vi "SST_Query.vi"(0 "System no.":i32=1 min=1 max=4 step=1, 2 "Axes to query":string[](array[string]), 3 "All axes?":bool, 4 "Axis identifier?":bool=TRUE, 5 "error in":errorcluster) -> (14 "Step size":dbl[](array[numeric]) format="%.6f", 19 "error out":errorcluster)   [LabVIEW 2020]
doc: "Returns step-size setting (e.g. for manual control pad, see also \"SST.vi\").\n\nC-702, C-867, C-880, E-871, E-873: If All axes = TRUE, then Axis identifier can be FALSE\n\nC-887, F-206, M-8X0: All axes = TRUE, Axis identifier = FALSE. Only values for axes X,Y,Z,U,V,W are valid"
panel:
  # "Returns step-size setting (e.g. for manual control pad, see also \"SST.vi\")."
  # "If all axes: use"
  # "Query"
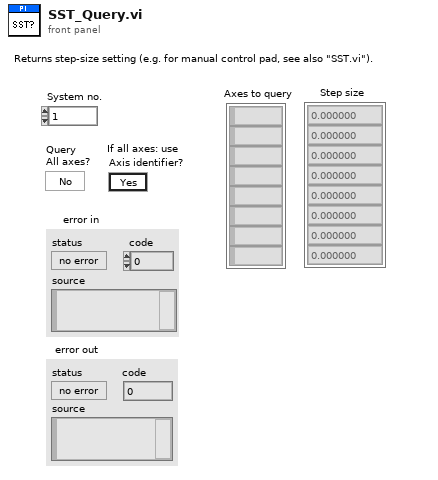
[diagram p1: front panel]
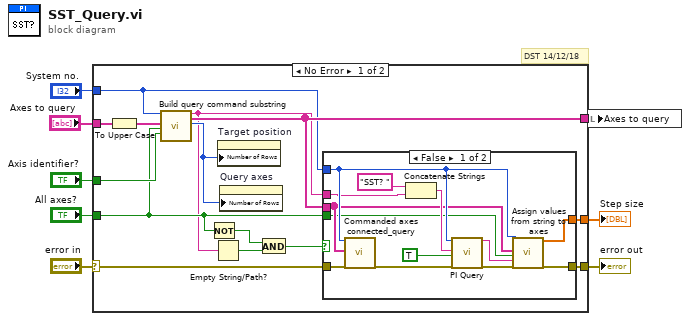
[diagram p0: block diagram]
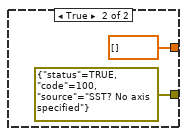
[diagram p2: hidden frame]
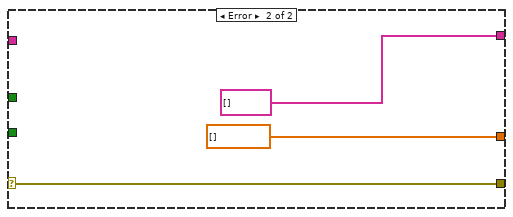
[diagram p3: hidden frame]
diagram:
  # "DST 14/12/18"
  n1 = case shown="No Error" "error in" {
    selector: "error in" -> [w10 w38]
    tunnel: [w22 dbl[] [] ("Values")] -> w8
    tunnel: "Axes to query" -> [w21 _]
    tunnel: [w20 w38] -> w6
    tunnel: "Axis identifier?" -> [w18 _]
    tunnel: "System no." -> [w9 _]
    tunnel: [w16 string[] [] ("Axes to query out")] -> w3
    tunnel: "All axes?" -> [w15 _]
    frame No Error {
      n2 = To Upper Case(1:w21) -> (0:w19:string[])
      n3 = call "Build query command substring.vi"("System no."=w9, "Axes to query in"=w19, "Query\nAll axes?"=w15, "For all axes: use\nAxis identifier?"=w18) -> ("Command substring"=w13:string, "Axes to query out"=w16:string[], "Number of rows"=w17:u32)  [unwired: 2 in, 11 out]
      n4 = Not(x=w15) -> (.not. x?=w14:bool)
      n5 = Empty String/Path?(string/path=w13) -> (empty?=w12:bool)
      n6 = property on="Target position" class="Arr (strict)"("Number of Rows"=w17) -> ()  [unwired: 2 in, 2 out]
      n7 = property on="Query axes" class="Arr (strict)"("Number of Rows"=w17) -> ()  [unwired: 2 in, 2 out]
      n8 = And(x=w14, y=w12) -> (x .and. y?=w11:bool)
      n9 = case shown="False" w11 {
        tunnel: [w32 dbl[] [] ("Values")] -> w22
        tunnel: w10 -> [w31 _]
        tunnel: [w27 errorcluster {"status"=TRUE, "code"=100, "source"="SST? No axis specified"} ("error out")] -> w20
        tunnel: w9 -> [w30 _]
        tunnel: w16 -> [w29 _]
        tunnel: w15 -> [w28 _]
        tunnel: w13 -> [w23 _]
        frame False {
          n10 = call "Commanded axes connected_query.vi"("System no."=w30, "Commanded axes"=w29, "error in"=w31) -> ("error out"=w26:errorcluster)  [unwired: 1 in, 15 out]
          n11 = Concatenate Strings("SST? ", w23) -> (w33:string)
          n12 = call "PI Query.vi"("System no."=w30, "String to send"=w33, "Attach termination char.?"=TRUE ("Attach Linefeed?"), "error in"=w26) -> ("String read"=w25:string, "error out"=w24:errorcluster)  [unwired: 3 in, 11 out]
          n13 = call "Assign values from string to axes.vi"("System no."=w30, "Queried axes"=w29, "All axes queried?"=w28, "Input String"=w25, "error in"=w24) -> ("Values"=w32:dbl[], "error out"=w27:errorcluster)  [unwired: 4 in, 9 out]
        }
        frame True {
        }
      }
    }
    frame Error {
    }
  }
  "error out" <- w6
  "Step size" <- w8
  n14 = local write "Axes to query"(w3) -> ()
